vi "String To Time.vi"(8 "error in (no error)":errorcluster, 10 "String Array In":string[](array[string])) -> (0 "error out":errorcluster, 2 "Time Stamp Out":timestamp[](array[timestamp]) format="%<%X>T")   [LabVIEW 2023]
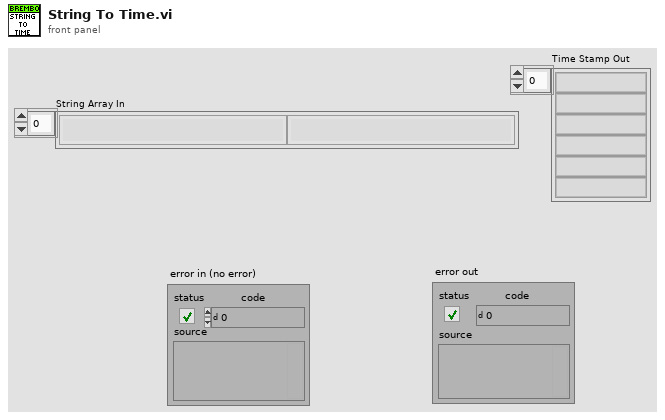
[diagram p1: front panel]
types:
  T1 = cluster{"second":i32, "minute":i32, "hour":i32, "day of month":i32, "month":i32, "year":i32, "day of week":i32, "day of year":i32, "is DST":i32}
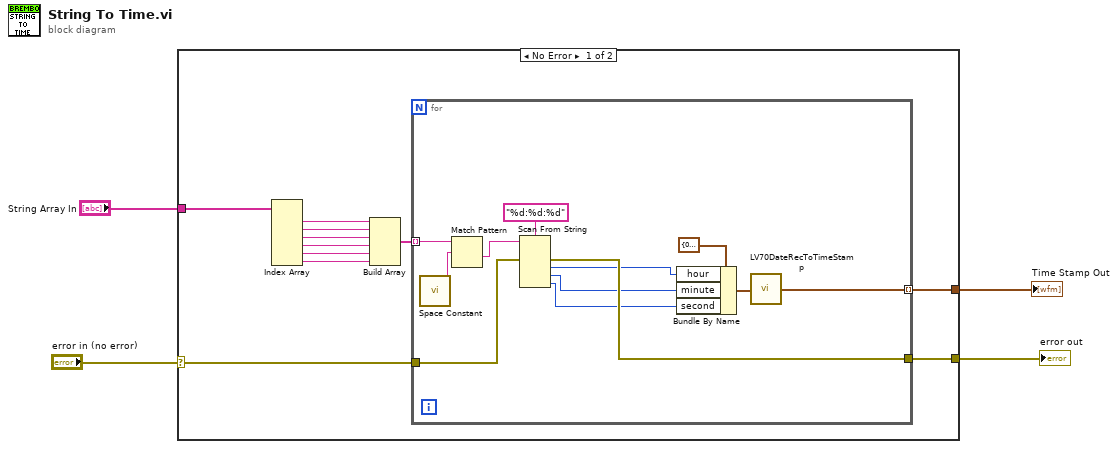
[diagram p0: block diagram]
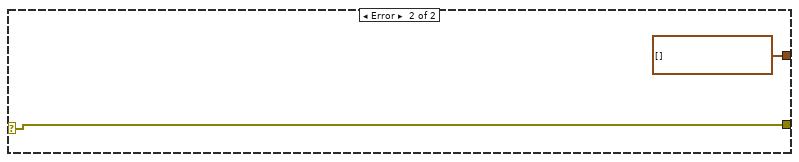
[diagram p2: hidden frame]
diagram:
  n1 = case shown="No Error" "error in (no error)" {
    selector: "error in (no error)" -> [w14 w29]
    tunnel: "String Array In" -> [w11 _]
    tunnel: [w15 timestamp[] []] -> w3
    tunnel: [w13 w29] -> w1
    frame No Error {
      n2 = Index Array(array=w11) -> (element #1=w10:string, element #2=w9:string, element #3=w8:string, element #4=w7:string, element #5=w6:string, element #6=w5:string)  [unwired: 6 in]
      n3 = Build Array(w10, w9, w8, w7, w6, w5) -> (w12:string[])
      n4 = for {
        tunnel: w12 -> [w22] mode=indexing
        tunnel: [w26] -> w15 mode=indexing
        tunnel: w14 -> [w25]
        tunnel: [w24] -> w13
        n5 = call <vilib>:"Space Constant.vi"() -> ("String"=w23:string)
        n6 = Match Pattern(string=w22, regular expression=w23) -> (after substring=w21:string)  [unwired: 1 in, 3 out]
        n7 = Scan From String(format string="%d:%d:%d", input string=w21, error in=w25) -> (error out=w24:errorcluster, output 1=w18:i32, output 2=w17:i32, output 3=w16:i32)  [unwired: 4 in, 2 out]
        n8 = Bundle By Name(cluster=T1 {"second"=0, "minute"=0, "hour"=0, "day of month"=1, "month"=1, "year"=2018, "day of week"=0, "day of year"=0, "is DST"=0} ("date time rec"), "hour"=w18, "minute"=w17, "second"=w16) -> (w20:T1)
        n9 = call <vilib>:"LV70DateRecToTimeStamp.vi"("date time rec"=w20) -> ("Time Stamp"=w26:timestamp)
      }
    }
    frame Error {
    }
  }
  "Time Stamp Out" <- w3
  "error out" <- w1
